vi "Convert Trajectory Data 4.0.vi"(1 "pre 4.0":T3(array[cluster])) -> (0 "post 4.0":T2(array[cluster]))   [LabVIEW 2025]
uses:
  Types/Segment Type.ctl
  Types/Trajectory Data.ctl
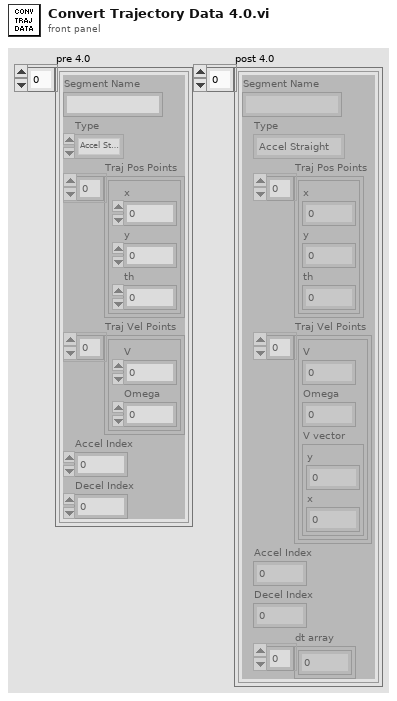
[diagram p1: front panel]
types:
  T1 = typedef "Segment Type.ctl" = enum16{"Accel Straight", "Const Straight", "Blend", "Circle", "Bezier", "Choreo"}
  T2 = cluster{"Segment Name":string, "Type":T1, "Traj Pos Points":cluster{"x":dbl, "y":dbl, "th":dbl}[], "Traj Vel Points":cluster{"V":dbl, "Omega":dbl, "V vector":cluster{"y":dbl, "x":dbl}}[], "Accel Index":i32, "Decel Index":i32, "dt array":dbl[]}[]
  T3 = cluster{"Segment Name":string, "Type":T1, "Traj Pos Points":cluster{"x":dbl, "y":dbl, "th":dbl}[], "Traj Vel Points":cluster{"V":dbl, "Omega":dbl}[], "Accel Index":i32, "Decel Index":i32}[]
  T4 = typedef "Trajectory Data.ctl" = cluster{"Segment Name":string, "Type":T1, "Traj Pos Points":cluster{"x":dbl, "y":dbl, "th":dbl}[], "Traj Vel Points":cluster{"V":dbl, "Omega":dbl, "V vector":cluster{"y":dbl, "x":dbl}}[], "Accel Index":i32, "Decel Index":i32}[]
  T5 = cluster{"Segment Name":string, "Type":T1, "Traj Pos Points":cluster{"x":dbl, "y":dbl, "th":dbl}[], "Traj Vel Points":cluster{"V":dbl, "Omega":dbl, "V vector":cluster{"y":dbl, "x":dbl}}[], "Accel Index":i32, "Decel Index":i32}
  T6 = cluster{"V":dbl, "Omega":dbl, "V vector":cluster{"y":dbl, "x":dbl}}[]
  T7 = cluster{"Segment Name":string, "Type":T1, "Traj Pos Points":cluster{"x":dbl, "y":dbl, "th":dbl}[], "Traj Vel Points":cluster{"V":dbl, "Omega":dbl, "V vector":cluster{"y":dbl, "x":dbl}}[], "Accel Index":i32, "Decel Index":i32, "dt array":dbl[]}
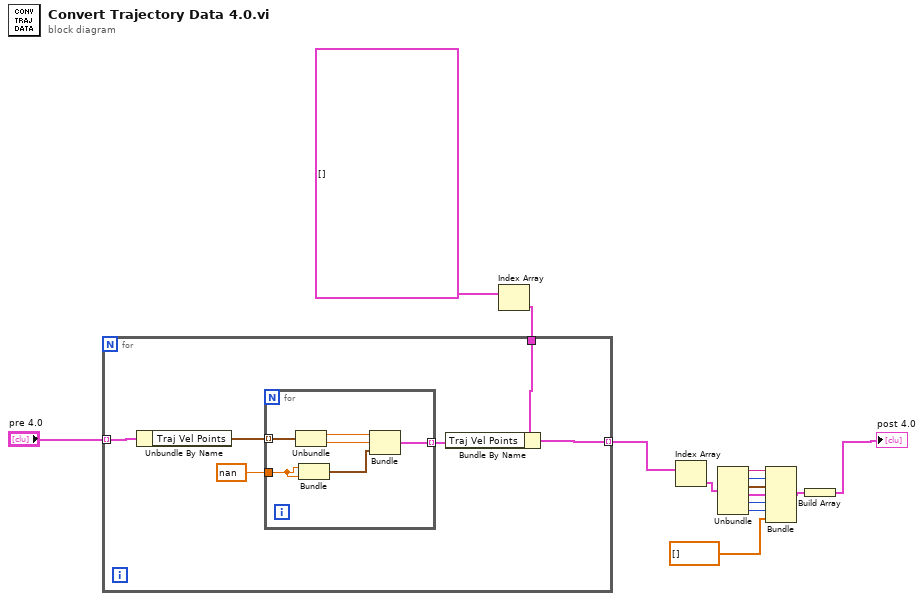
[diagram p0: block diagram]
diagram:
  n1 = Index Array(array=T4 [] ("post 4.0")) -> (element=w12:T5)  [unwired: 1 in]
  n2 = for {
    tunnel: "pre 4.0" -> [w20] mode=indexing
    tunnel: w12 -> [w19]
    tunnel: [w15] -> w2 mode=indexing
    n3 = Unbundle By Name(w20) -> ("Traj Vel Points"=w18:cluster{"V":dbl, "Omega":dbl}[])
    n4 = for {
      tunnel: w18 -> [w26] mode=indexing
      tunnel: nan -> [w25]
      tunnel: [w21] -> w16 mode=indexing
      n5 = Unbundle(w26) -> ("V"=w24:dbl, "Omega"=w23:dbl)
      n6 = Bundle(w25, w25) -> (w22:cluster{dbl, dbl})  [unwired: 1 in]
      n7 = Bundle("V"=w24, "Omega"=w23, w22) -> (w21:cluster{"V":dbl, "Omega":dbl, cluster{dbl, dbl}})  [unwired: 1 in]
    }
    n8 = Bundle By Name(cluster=w19, "Traj Vel Points"=w16) -> (w15:T5)
  }
  n9 = Index Array(array=w2) -> (element=w11:T5)  [unwired: 1 in]
  n10 = Unbundle(w11) -> ("Segment Name"=w10:string, "Type"=w9:T1, "Traj Pos Points"=w8:cluster{"x":dbl, "y":dbl, "th":dbl}[], "Traj Vel Points"=w7:T6, "Accel Index"=w6:i32, "Decel Index"=w5:i32)
  n11 = Bundle("Segment Name"=w10, "Type"=w9, "Traj Pos Points"=w8, "Traj Vel Points"=w7, "Accel Index"=w6, "Decel Index"=w5, "dt array"=dbl[] []) -> (w3:T7)  [unwired: 1 in]
  n12 = Build Array(w3) -> (→"post 4.0":T2)
